vi "Init CVT.vi"(8 "error in":errorcluster, 11 "Controller in":refnum<class "Controller.lvclass">) -> (0 "error out":errorcluster, 3 "Controller out":refnum<class "Controller.lvclass">)   [LabVIEW 2014, in "Controller.lvlib" / "Controller.lvclass"]
uses:
  Controller.lvclass
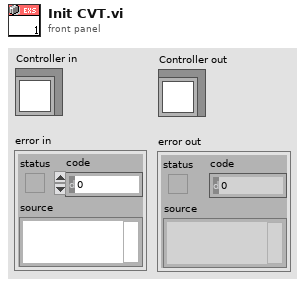
[diagram p1: front panel]
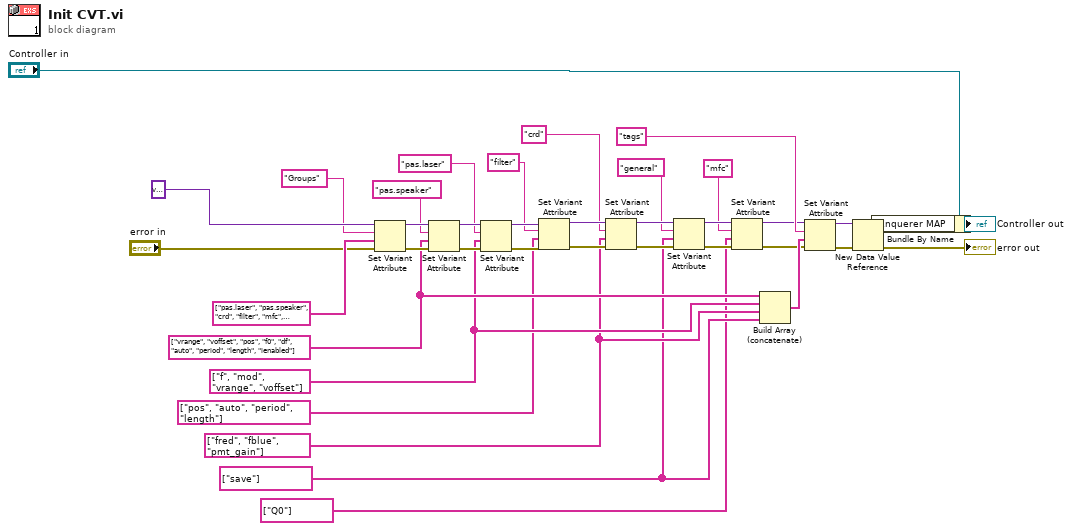
[diagram p0: block diagram]
diagram:
  w7 = string[] ["save"]
  w18 = string[] ["fred", "fblue", "pmt_gain"]
  w20 = string[] ["f", "mod", "vrange", "voffset"]
  w21 = string[] ["vrange", "voffset", "pos", "f0", "df", "auto", "period", "length", "ienabled"]
  n1 = Set Variant Attribute(Variant=variant ("variant"), name="Groups", value=string[] ["pas.laser", "pas.speaker", "crd", "filter", "mfc", "general"], error in="error in") -> (Variant out=w35:variant, error out=w34:errorcluster)  [unwired: 1 out]
  n2 = Set Variant Attribute(Variant=w35, name="pas.speaker", value=w21, error in=w34) -> (Variant out=w32:variant, error out=w31:errorcluster)  [unwired: 1 out]
  n3 = Set Variant Attribute(Variant=w32, name="pas.laser", value=w20, error in=w31) -> (Variant out=w27:variant, error out=w28:errorcluster)  [unwired: 1 out]
  n4 = Set Variant Attribute(Variant=w27, name="filter", value=string[] ["pos", "auto", "period", "length"], error in=w28) -> (Variant out=w25:variant, error out=w24:errorcluster)  [unwired: 1 out]
  n5 = Set Variant Attribute(Variant=w25, name="crd", value=w18, error in=w24) -> (Variant out=w9:variant, error out=w10:errorcluster)  [unwired: 1 out]
  n6 = Set Variant Attribute(Variant=w9, name="general", value=w7, error in=w10) -> (Variant out=w5:variant, error out=w6:errorcluster)  [unwired: 1 out]
  n7 = Set Variant Attribute(Variant=w5, name="mfc", value=string[] ["Q0"], error in=w6) -> (Variant out=w3:variant, error out=w2:errorcluster)  [unwired: 1 out]
  n8 = Build Array (concatenate)(w21, w20, w18, w7) -> (w17:string[])
  n9 = Set Variant Attribute(Variant=w3, name="tags", value=w17, error in=w2) -> (Variant out=w15:variant, error out=w16:errorcluster)  [unwired: 1 out]
  n10 = New Data Value Reference(data value=w15, error in=w16) -> (data value reference=w12:refnum<data-value>, error out=→"error out":errorcluster)
  n11 = Bundle By Name(cluster="Controller in", "Enquerer MAP"=w12) -> (→"Controller out":refnum<class "Controller.lvclass">)
